vi "Zadanie6.vi"() -> ()   [LabVIEW 2011]
panel:
  out "Waveform Chart":dbl(graph)
  out "Tank":dbl(slide) scale=0.0..20.0
  in  "stop":bool
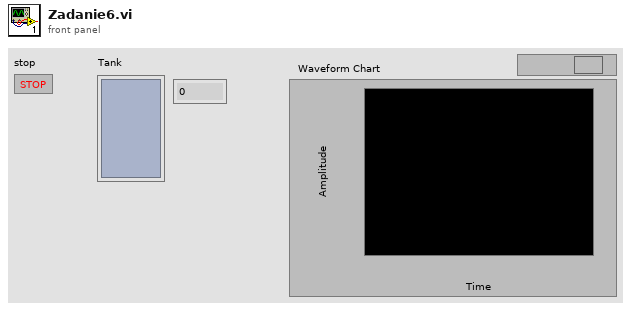
[diagram p1: front panel]
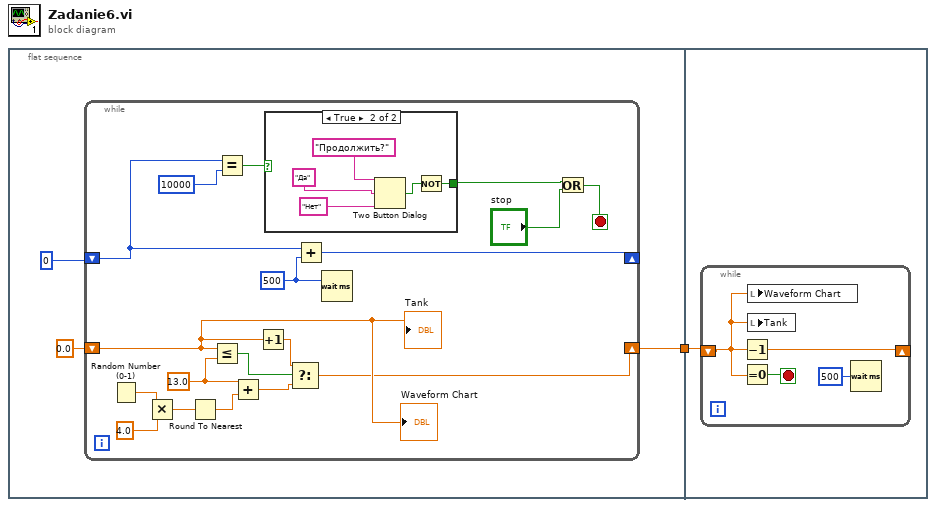
[diagram p0: block diagram]
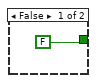
[diagram p2: hidden frame]
diagram:
  n1 = flat-sequence {
    tunnel: [w2] -> w1
    tunnel: w1 -> [w29]
    frame #0 {
      n2 = while {
        shift-right: [w14] -> w2
        shift-left: 0.0 -> [w15]
        shift-right: [w8] -> _
        shift-left: 0 -> [w9]
        stop <- w7 stop-if-true
        w10 = 500
        w18 = 13.0
        n3 = Random Number (0-1)() -> (number: 0 to 1=w16:dbl)
        n4 = Multiply(x=w16, y=4.0) -> (x*y=w22:dbl)
        n5 = Round To Nearest(number=w22) -> (nearest integer value=w21:dbl)
        n6 = Less Or Equal?(x=w15, y=w18) -> (x <= y?=w13:bool)
        n7 = Equal?(x=w9, y=10000) -> (x = y?=w11:bool)
        n8 = Add(x=w18, y=w21) -> (x+y=w20:dbl)
        n9 = Increment(x=w15) -> (x+1=w19:dbl)
        n10 = case shown="True" w11 {
          tunnel: [FALSE w24] -> w5
          frame False {
          }
          frame True {
            n11 = Two Button Dialog(message="Продолжить?", 1:"Нет", 2:"Да") -> (T button?=w25:bool)
            n12 = Not(x=w25) -> (.not. x?=w24:bool)
          }
        }
        n13 = Select(t=w19, s=w13, f=w20) -> (s? t:f=w14:dbl)
        n14 = Add(x=w9, y=w10) -> (x+y=w8:i32)
        n15 = Wait (ms)(milliseconds to wait=w10) -> ()  [unwired: 1 out]
        n16 = Or(x=w5, y="stop") -> (x .or. y?=w7:bool)
        "Tank" <- w15
        "Waveform Chart" <- w15
      }
    }
    frame #1 {
      n17 = while {
        shift-right: [w30] -> _
        shift-left: w29 -> [w33]
        stop <- w32 stop-if-true
        n18 = Decrement(x=w33) -> (x-1=w30:dbl)
        n19 = Equal To 0?(x=w33) -> (x = 0?=w32:bool)
        n20 = local write "Waveform Chart"(w33) -> ()
        n21 = local write "Tank"(w33) -> ()
        n22 = Wait (ms)(milliseconds to wait=500) -> ()  [unwired: 1 out]
      }
    }
  }
